vi "test.copy all.vi"(8 "error in (no error)":errorcluster, 11 "TestCase in":refnum<class "TestCase.Pointer.lvclass">) -> (0 "error out":errorcluster, 3 "TestCase out":refnum<class "TestCase.Pointer.lvclass">)   [LabVIEW 2016, in "TestCase.Pointer.lvclass"]
uses:
  TestCase.Pointer.lvclass
  TestCase.Pointer.lvclass/TestCase.Pointer.ctl
  <vilib>/addons/_JKI Toolkits/VI Tester/TestCase.llb/TestCase.lvclass
  Source/Classes/Pointer/Pointer.lvclass
  C:/Program Files (x86)/National Instruments/LabVIEW 2016/vi.lib/addons/_JKI Toolkits/VI Tester/TestCase.llb/TestCase.lvclass
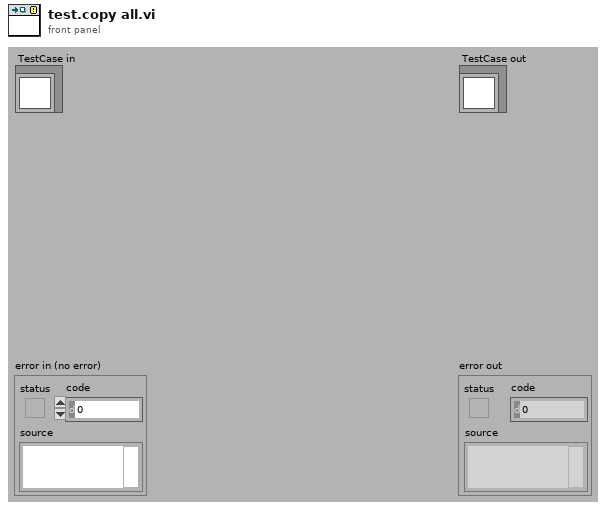
[diagram p1: front panel]
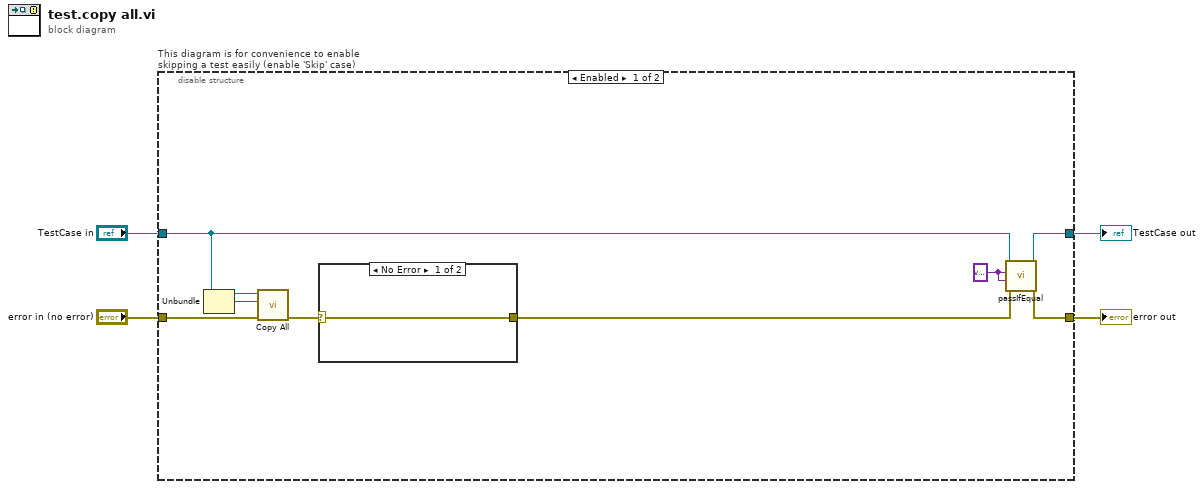
[diagram p0: block diagram]
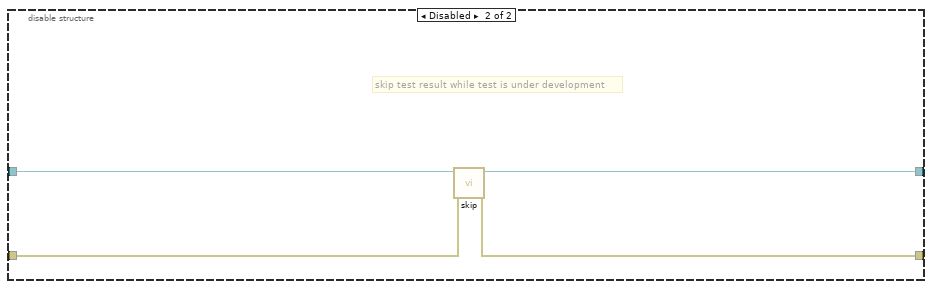
[diagram p3: hidden frame]
diagram:
  n1 = disable-structure "This diagram is for convenience to enable skipping a test easily (enable 'Skip' case)" shown="Enabled" {
    disable-tunnel: "TestCase in" -> [w11 w19]
    disable-tunnel: [w13 w17] -> w1
    disable-tunnel: [w12 w18] -> w3
    disable-tunnel: "error in (no error)" -> [w7 w16]
    frame Enabled {
      w10 = variant ("x")
      n2 = Unbundle(w11) -> (w9:refnum<class "Pointer.lvclass">, w8:refnum<class "Pointer.lvclass">)  [unwired: 1 out]
      n3 = call "Copy All.vi"("error in (no error)"=w7, "dst Pointer in"=w8, "src Pointer in"=w9) -> ("error out"=w6:errorcluster)  [unwired: 6 in, 2 out]
      n4 = case shown="No Error" w6 {
        selector: w6 -> [w14 w15]
        tunnel: [w14 w15] -> w5
        frame No Error {
        }
        frame Error {
        }
      }
      n5 = call-dynamic "passIfEqual.vi"("error in (no error)"=w5, "y"=w10, "x"=w10, "TestCase in"=w11) -> ("error out"=w12:errorcluster, "TestCase out"=w13:refnum<class "TestCase.Pointer.lvclass">)  [unwired: 6 in]
    }
    frame Disabled {
      # "skip test result while test is under development"
      n6 = call <vilib>:"skip.vi"("error in (no error)"=w16, "TestCase in"=w19) -> ("error out"=w18:errorcluster, "TestCase out"=w17:refnum<class "TestCase.Pointer.lvclass">)  [unwired: 8 in]
    }
  }
  "error out" <- w3
  "TestCase out" <- w1
